vi "TesterXML.vi"() -> ()   [LabVIEW 2014]
uses:
  NationalInstruments.VeriStand.XMLReader
  <vilib>/Utility/sysdir.llb/System Directory Type.ctl
  CEF Sandbox/Configuration Tool.lvlib
panel:
  out "path":path
  out "Source.Path Type 2":T1(ring)
  in  "Source.Path Type":T1(ring)
  in  "Path In":path
  out "NaN/Path/Refnum?":bool
  out "TimingSource":refnum<k24>
  out "error":string
  in  "error in":errorcluster
  in  "selected path":path=path "C:/Users/Public/Documents/National Instruments/NI VeriStand 2014/Custom Devices/Scan Engine/Custom Device Scan Engine.xml"
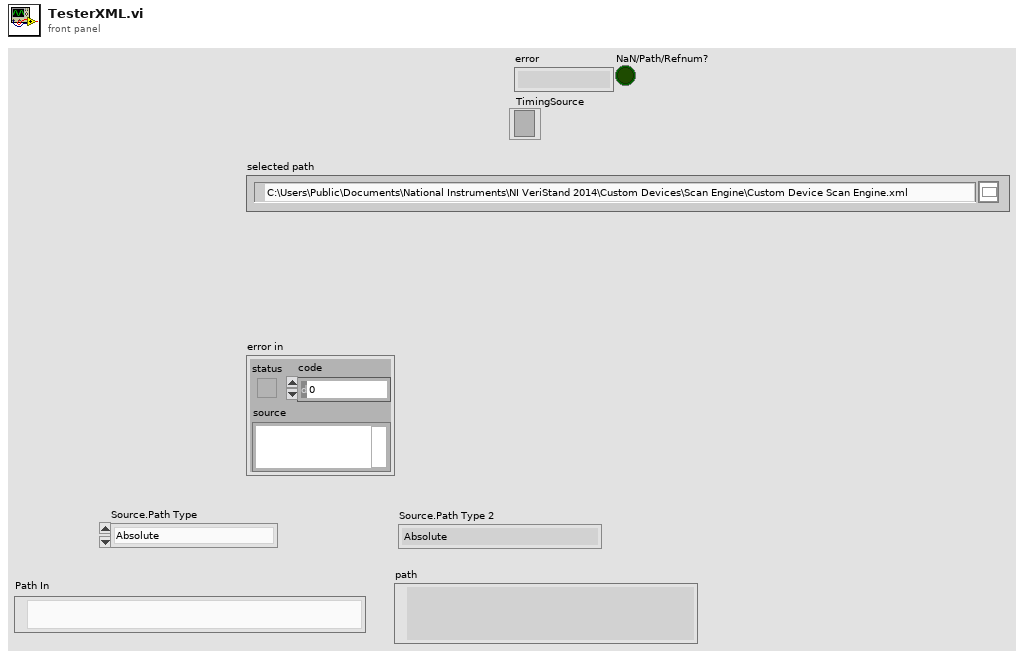
[diagram p1: front panel]
types:
  T1 = enum16{"Absolute", "To Base", "To Common Doc Dir", "To Application Data Dir"}
  T2 = typedef "System Directory Type.ctl" = i32
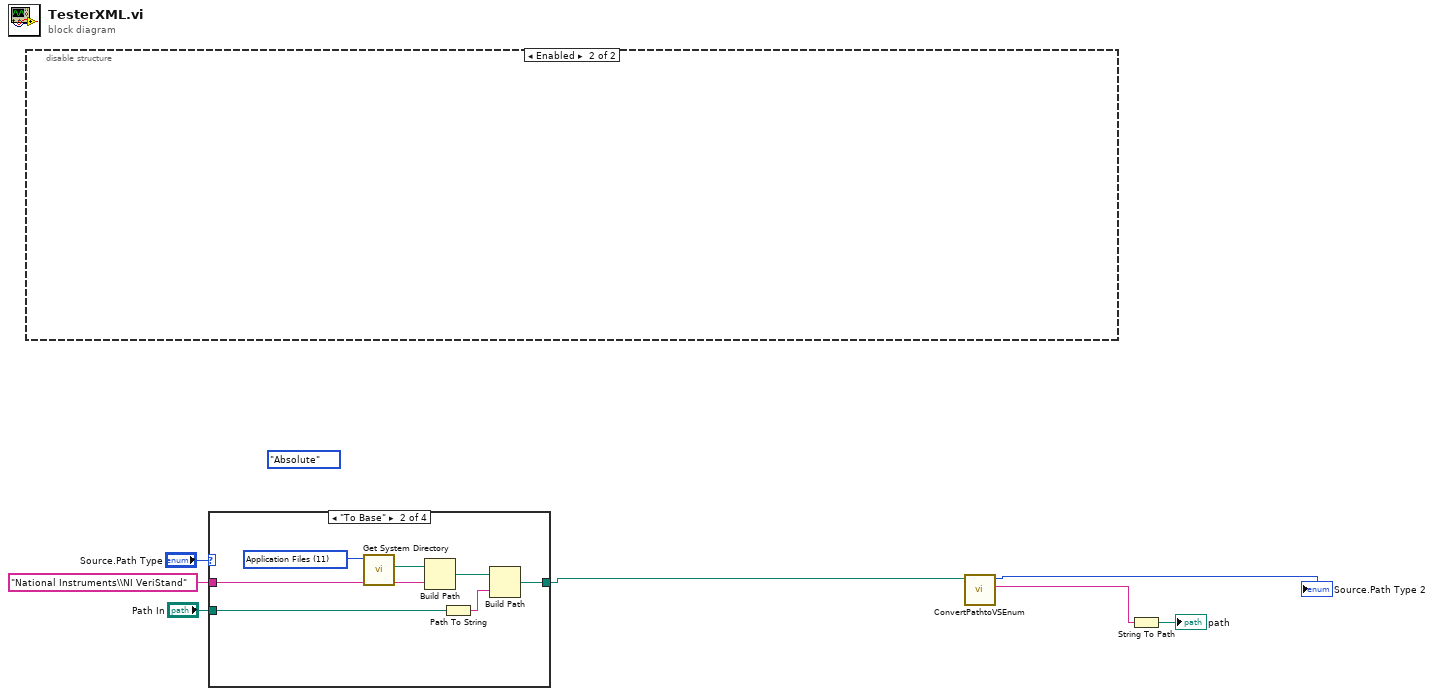
[diagram p0: block diagram]
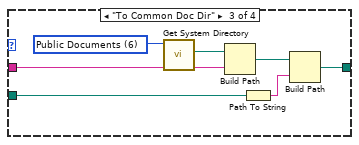
[diagram p3: hidden frame]
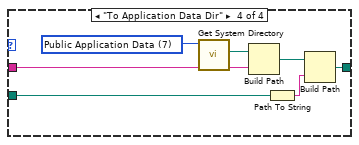
[diagram p4: hidden frame]
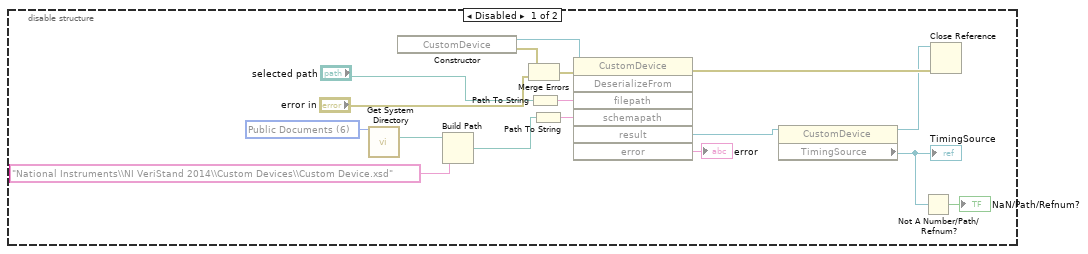
[diagram p5: hidden frame]
diagram:
  (unwired) T1."Absolute" ("Source.Path Type")
  n1 = disable-structure shown="Enabled" {
    frame Disabled {
      w15 = T2 6 items=["User Home"=0, "User Desktop"=1, "User Documents"=2, "User Application Data"=3, "User Preferences"=4, "User Temporary"=5, "Public Documents"=6, "Public Application Data"=7, "Public Preferences"=8, "Public Cache"=13, "System Core Libraries"=9, "System Installed Libraries"=10, "Application Files"=11, "Boot Volume Root"=12] ("system directory type")
      n2 = call <vilib>:"Get System Directory.vi"("system directory type"=w15) -> ("system directory"=w16:path)  [unwired: 10 in]
      n3 = constructor class="CustomDevice"() -> (reference out=w20:refnum<k24>, error out=w23:errorcluster)  [unwired: 3 in, 1 out]
      n4 = Build Path(base path=w16, name or relative path="National Instruments\\NI VeriStand 2014\\Custom Devices\\Custom Device.xsd") -> (appended path=w14:path)
      n5 = Merge Errors(w23, "error in") -> (w24:errorcluster)
      n6 = Path To String(path="selected path") -> (string=w21:string)
      n7 = Path To String(path=w14) -> (string=w22:string)
      n8 = invoke class="CustomDevice" method="DeserializeFrom"(reference=w20, error in=w24, "filepath"=w21, "schemapath"=w22) -> (error out=w13:errorcluster, "result"=w11:refnum<k24>, "error"=→"error":string)  [unwired: 3 in, 4 out]
      n9 = property class="CustomDevice"(reference=w11) -> (reference out=w10:refnum<k24>, "TimingSource"=w9:refnum<k24>)  [unwired: 1 in, 1 out]
      "TimingSource" <- w9
      n10 = Not A Number/Path/Refnum?(number/path/refnum=w9) -> (NaN/Path/Refnum?=→"NaN/Path/Refnum?":bool)
      n11 = Close Reference(reference=w10, error in (no error)=w13) -> ()  [unwired: 1 out]
    }
    frame Enabled {
    }
  }
  n12 = case shown="\"To Base\"" "Source.Path Type" {
    tunnel: "Path In" -> [w25 w28 w35 w42]
    tunnel: [w25 w27 w34 w41] -> w4
    tunnel: "National Instruments\\NI VeriStand" ("name or relative path") -> [_ w26 w33 w40]
    frame "Absolute", Default {
    }
    frame "To Base" {
      w32 = T2 11 items=["User Home"=0, "User Desktop"=1, "User Documents"=2, "User Application Data"=3, "User Preferences"=4, "User Temporary"=5, "Public Documents"=6, "Public Application Data"=7, "Public Preferences"=8, "Public Cache"=13, "System Core Libraries"=9, "System Installed Libraries"=10, "Application Files"=11, "Boot Volume Root"=12] ("system directory type")
      n13 = call <vilib>:"Get System Directory.vi"("system directory type"=w32) -> ("system directory"=w31:path)  [unwired: 10 in]
      n14 = Build Path(base path=w31, name or relative path=w26) -> (appended path=w30:path)
      n15 = Path To String(path=w28) -> (string=w29:string)
      n16 = Build Path(base path=w30, name or relative path=w29) -> (appended path=w27:path)
    }
    frame "To Common Doc Dir" {
      w39 = T2 6 items=["User Home"=0, "User Desktop"=1, "User Documents"=2, "User Application Data"=3, "User Preferences"=4, "User Temporary"=5, "Public Documents"=6, "Public Application Data"=7, "Public Preferences"=8, "Public Cache"=13, "System Core Libraries"=9, "System Installed Libraries"=10, "Application Files"=11, "Boot Volume Root"=12] ("system directory type")
      n17 = call <vilib>:"Get System Directory.vi"("system directory type"=w39) -> ("system directory"=w38:path)  [unwired: 10 in]
      n18 = Build Path(base path=w38, name or relative path=w33) -> (appended path=w37:path)
      n19 = Path To String(path=w35) -> (string=w36:string)
      n20 = Build Path(base path=w37, name or relative path=w36) -> (appended path=w34:path)
    }
    frame "To Application Data Dir" {
      w46 = T2 7 items=["User Home"=0, "User Desktop"=1, "User Documents"=2, "User Application Data"=3, "User Preferences"=4, "User Temporary"=5, "Public Documents"=6, "Public Application Data"=7, "Public Preferences"=8, "Public Cache"=13, "System Core Libraries"=9, "System Installed Libraries"=10, "Application Files"=11, "Boot Volume Root"=12] ("system directory type")
      n21 = call <vilib>:"Get System Directory.vi"("system directory type"=w46) -> ("system directory"=w45:path)  [unwired: 10 in]
      n22 = Build Path(base path=w45, name or relative path=w40) -> (appended path=w44:path)
      n23 = Path To String(path=w42) -> (string=w43:string)
      n24 = Build Path(base path=w44, name or relative path=w43) -> (appended path=w41:path)
    }
  }
  n25 = call "ConvertPathtoVSEnum.vi"("Path In"=w4) -> ("Remaining Path"=w2:string, "VS Enum Out"=→"Source.Path Type 2":T1)  [unwired: 9 in]
  n26 = String To Path(string=w2) -> (path=→"path":path)
